vi "GetSensorValues.vi"(1 "Ref_BuiltInAccelerometer":T3={"DevStatus"={"status"=FALSE, "code"=0, "source"=""}, "Scaling"={"Gain (VoltsPerG)"=0.0, "Center Voltage"=0.0}, "Analog Channels"={"X-Axis"=enum."Invalid", "Y-Axis"=enum."Invalid", "Z-Axis"=enum."Invalid"}, "I2C Bus"=enum."Invalid", "SPI Bus"=enum."Invalid", "Accel Range"=0, "ADXL Axes"={"X-Axis"=FALSE, "Y-Axis"=FALSE, "Z-Axis"=FALSE}, "Handle"=0, "Device Address"=0, "Accel Type"=enum."Analog"} {"Device Address" format="%.0x"; "Accel Range" items=["+/- 2 g", "+/- 4 g", "+/- 8 g", "+/- 16 g"]}, 3 "Rear Prox Sensor":T1, 4 "Right Prox Sensor":T1, 5 "Left Prox Sensor":T1, 6 "Upper Pressure Transducer":T1, 8 "Ref_Compressor":T15, 9 "Front-Right Prox Sensor":T1, 10 "Ref_ElevatorEncoder":T10={"DeviceStatus"={"status"=FALSE, "code"=0, "source"=""}, "Type"=enum."PWM", "PWM"={"PWM Channel"=enum."Invalid", "DeadBand"={"Name"="", "maxPositivePwm"=0, "minPositivePwm"=0, "centerPwm"=0, "maxNegativePwm"=0, "minNegativePwm"=0, "angularRange"=0}}, "CAN"={"Device Number"=0, "SetOutput VI Ref"=variant, "GetOutput VI Ref"=variant, "Enable VI Ref"=variant, "Disable VI Ref"=variant, "Data"=variant}, "Invert"=FALSE, "DIO PWM"={"PWM \"Enable\" Channel"=enum."Invalid", "DIOChannel"=enum."Invalid", "PWM Rate"=0.0}}, 11 "Front-Left Prox Sensor":T1, 12 "Ref_ElevatorLimitSwitches":T10={"DeviceStatus"={"status"=FALSE, "code"=0, "source"=""}, "Type"=enum."PWM", "PWM"={"PWM Channel"=enum."Invalid", "DeadBand"={"Name"="", "maxPositivePwm"=0, "minPositivePwm"=0, "centerPwm"=0, "maxNegativePwm"=0, "minNegativePwm"=0, "angularRange"=0}}, "CAN"={"Device Number"=0, "SetOutput VI Ref"=variant, "GetOutput VI Ref"=variant, "Enable VI Ref"=variant, "Disable VI Ref"=variant, "Data"=variant}, "Invert"=FALSE, "DIO PWM"={"PWM \"Enable\" Channel"=enum."Invalid", "DIOChannel"=enum."Invalid", "PWM Rate"=0.0}}, 15 "Tank Pressure Transducer":T1, 19 "Ground Prox Sensor":T1, 20 "Ref_Drive 1R":T10, 21 "Ref_Drive 2R":T10, 22 "Ref_Drive 3L":T10, 23 "Ref_Drive 4L":T10) -> ()   [LabVIEW 2018]
uses:
  <vilib>/Rock Robotics/WPI/AnalogChannel/WPI_AnalogChannelDevRef.ctl
  <vilib>/Rock Robotics/SystemInterfaces/AI/FPGA_AIChannel.ctl
  <vilib>/Rock Robotics/WPI/Compressor/WPI_CompressorDevRef.ctl
  <vilib>/Rock Robotics/WPI/MotorControl/WPI_MotorControlDeviceRef.ctl
  <vilib>/Rock Robotics/WPI/MotorControl/WPI_MotorControlType.ctl
  <vilib>/Rock Robotics/SystemInterfaces/DIO/FPGA_DIOPWMChannel.ctl
  <vilib>/Rock Robotics/WPI/PWM/WPI_PWMDeadband.ctl
  <vilib>/Rock Robotics/SystemInterfaces/DIO/FPGA_DIOChannel.ctl
  <vilib>/Rock Robotics/WPI/Accelerometer/WPI_AccelerometerDevRef.ctl
  <vilib>/Rock Robotics/WPI/Accelerometer/WPI_AccelerometerScaling.ctl
  <vilib>/Rock Robotics/WPI/Accelerometer/WPI_AccelerometerAnalogChannels.ctl
  <vilib>/Rock Robotics/SystemInterfaces/i2clib/i2c_bus.ctl
  <vilib>/Rock Robotics/SystemInterfaces/spilib/spi_bus.ctl
  <vilib>/Rock Robotics/WPI/Accelerometer/ADXL345 Range.ctl
  <vilib>/Rock Robotics/WPI/Accelerometer/WPI_AccelerometerADXL345 Axes.ctl
  SensorReadings.vi
  RefNums_Actuators.vi
  RobotStates.vi
  Inputs_DriverStation.vi
  <vilib>/Rock Robotics/WPI/ThirdParty/Phoenix-LabVIEW/Motor Controller/Get/CTRE_Phoenix_MotorController_GetLimitSwitchStates.vi
  <vilib>/Rock Robotics/WPI/ThirdParty/Phoenix-LabVIEW/Motor Controller/Get/CTRE_Phoenix_MotorController_GetSelectedSensorData.vi
  <vilib>/gmath/NI_Gmath.lvlib
  <vilib>/Analysis/NI_AALBase.lvlib
panel:
  in  "Normal Elevator Std (A)":dbl=35.0
  in  "Off Ground Time (ms)":u32=100
  in  "On Ground Time (ms)":u32=1000
  in  "Ground Distance (in)":dbl=6.0
  in  "Plot Drive Encoder Data":bool
  in  "Tank Pressure Voltage Table":dbl[](array[numeric])=[0.4, 0.7, 0.9, 1.2, 1.4, 1.7, 1.9, 2.3, 2.5, 2.8, 3.0, 3.3] format="%_6g"
  in  "Tank Pressure PSI Table":dbl[](array[numeric])=[0.0, 10.0, 20.0, 30.0, 40.0, 50.0, 60.0, 70.0, 80.0, 90.0, 100.0, 115.0] format="%_6g"
  in  "LR Voltage Table":dbl[](array[numeric])=[0.43, 0.45, 0.47, 0.55, 0.6, 0.68, 0.72, 0.81, 0.86, 0.98, 1.13, 1.36, 1.53, 1.77, 1.99, 2.26, 2.52, 2.76] format="%_6g"
  in  "LR Distance Table":dbl[](array[numeric])=[150.661, 140.6, 133.7, 120.9, 110.1, 95.3, 90.1, 80.0, 73.7, 64.6, 55.9, 45.6, 40.2, 35.0, 29.6, 24.3, 19.6, 14.8] format="%_6g"
  in  "Suction Threshold (V)":dbl=0.15
  in  "SR Voltage Table":dbl[](array[numeric])=[3.15, 2.82, 2.51, 2.16, 1.92, 1.7, 1.49, 1.3, 1.12, 0.97, 0.87, 0.79, 0.72, 0.64, 0.61, 0.58, 0.52, 0.47, 0.46, 0.45, 0.43, 0.41] format="%_6g"
  in  "SR Distance Table":dbl[](array[numeric])=[4.6, 6.6, 8.3, 10.4, 12.2, 14.1, 16.5, 19.9, 23.6, 28.2, 32.6, 36.8, 40.9, 46.3, 49.9, 53.7, 58.3, 63.5, 67.5, 71.5, 75.1, 78.9] format="%_6g"
  out "Drive Encoder Velocities":cluster{dbl, dbl}(graph)
  # "*** Alpha was set to 6 inches ***"
  # "*** Beta was set to 12 inches ***"
  # "ADXL"
  # "Analog"
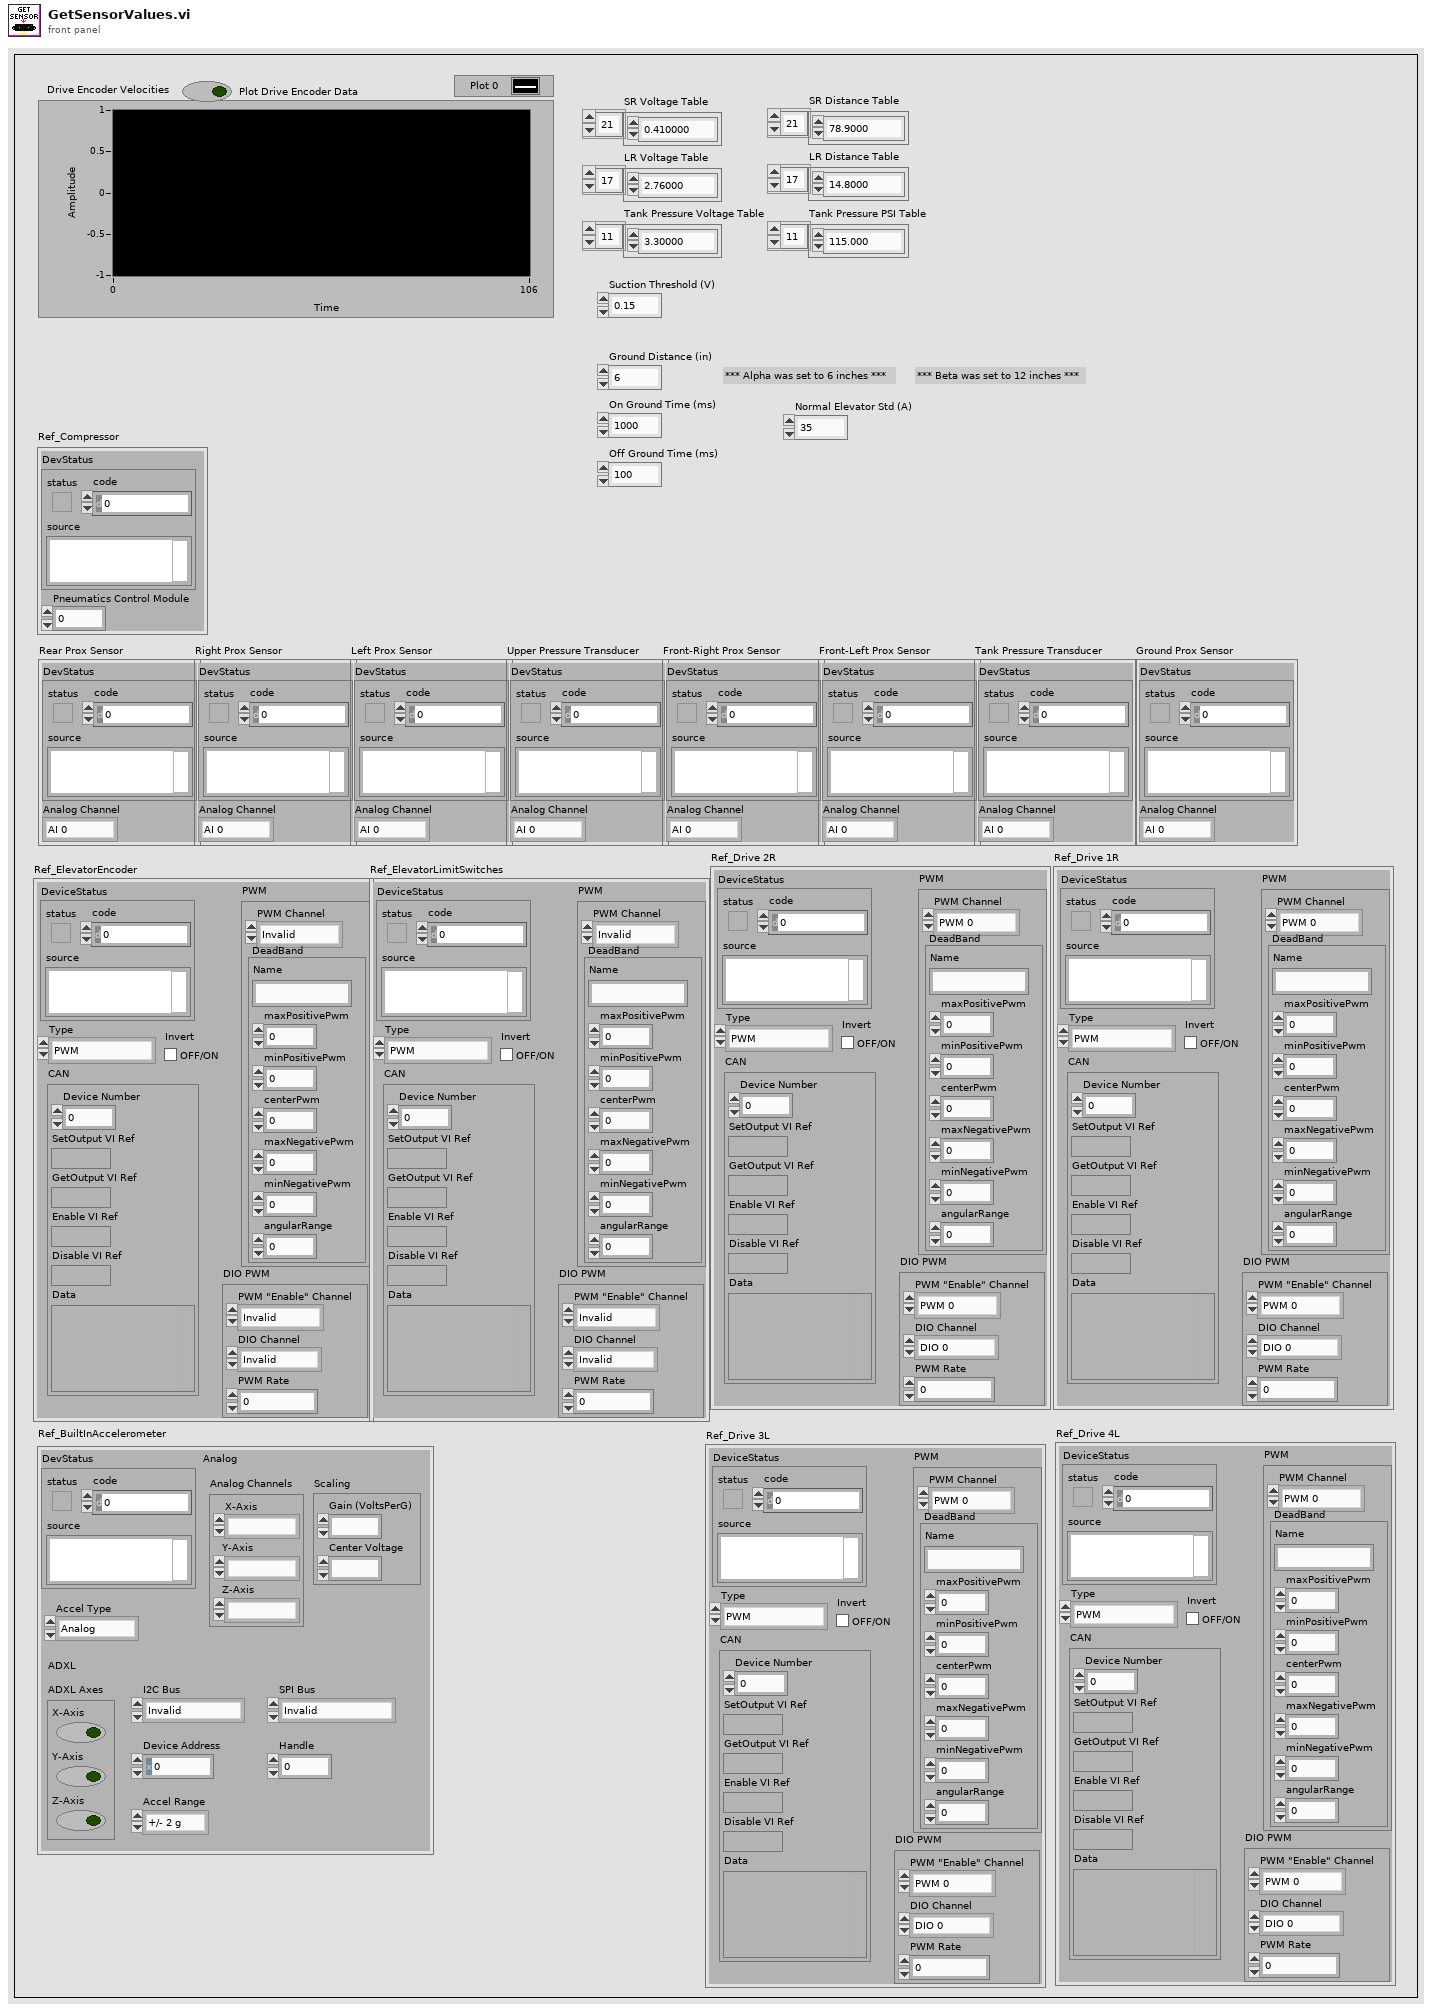
[diagram p1: front panel]
types:
  T1 = typedef "WPI_AnalogChannelDevRef.ctl" = cluster{"DevStatus":errorcluster, "Analog Channel":T2}
  T2 = typedef "FPGA_AIChannel.ctl" = enum8{"AI 0", "AI 1", "AI 2", "AI 3", "AI MXP 0", "AI MXP 1", "AI MXP 2", "AI MXP 3", "Invalid"}
  T3 = typedef "WPI_AccelerometerDevRef.ctl" = cluster{"DevStatus":errorcluster, "Scaling":T4, "Analog Channels":T5, "I2C Bus":T6, "SPI Bus":T7, "Accel Range":T8, "ADXL Axes":T9, "Handle":i32, "Device Address":u8, "Accel Type":enum16{"Analog", "ADXL345 I2C", "ADXL345 SPI", "Internal", "ADXL362 SPI"}}
  T4 = typedef "WPI_AccelerometerScaling.ctl" = cluster{"Gain (VoltsPerG)":dbl, "Center Voltage":dbl}
  T5 = typedef "WPI_AccelerometerAnalogChannels.ctl" = cluster{"X-Axis":T2, "Y-Axis":T2, "Z-Axis":T2}
  T6 = typedef "i2c_bus.ctl" = enum16{"I2C On-Board", "I2C MXP", "Invalid"}
  T7 = typedef "spi_bus.ctl" = enum16{"SPI On-Board, CS0", "SPI On-Board, CS1", "SPI On-Board, CS2", "SPI On-Board, CS3", "SPI MXP", "Invalid"}
  T8 = typedef "ADXL345 Range.ctl" = u8
  T9 = typedef "WPI_AccelerometerADXL345 Axes.ctl" = cluster{"X-Axis":bool, "Y-Axis":bool, "Z-Axis":bool}
  T10 = typedef "WPI_MotorControlDeviceRef.ctl" = cluster{"DeviceStatus":errorcluster, "Type":T11, "PWM":cluster{"PWM Channel":T12, "DeadBand":T13}, "CAN":cluster{"Device Number":u8, "SetOutput VI Ref":variant, "GetOutput VI Ref":variant, "Enable VI Ref":variant, "Disable VI Ref":variant, "Data":variant}, "Invert":bool, "DIO PWM":cluster{"PWM \"Enable\" Channel":T12, "DIOChannel":T14, "PWM Rate":dbl}}
  T11 = typedef "WPI_MotorControlType.ctl" = enum16{"PWM", "CAN", "DIO PWM"}
  T12 = typedef "FPGA_DIOPWMChannel.ctl" = enum8{"PWM 0", "PWM 1", "PWM 2", "PWM 3", "PWM 4", "PWM 5", "PWM 6", "PWM 7", "PWM 8", "PWM 9", "PWM MXP 0", "PWM MXP 1", "PWM MXP 2", "PWM MXP 3", "PWM MXP 4", "PWM MXP 5", "PWM MXP 6", "PWM MXP 7", "PWM MXP 8", "PWM MXP 9", "Invalid"}
  T13 = typedef "WPI_PWMDeadband.ctl" = cluster{"Name":string, "maxPositivePwm":i32, "minPositivePwm":i32, "centerPwm":i32, "maxNegativePwm":i32, "minNegativePwm":i32, "angularRange":u16}
  T14 = typedef "FPGA_DIOChannel.ctl" = enum8{"DIO 0", "DIO 1", "DIO 2", "DIO 3", "DIO 4", "DIO 5", "DIO 6", "DIO 7", "DIO 8", "DIO 9", "DIO MXP 0", "DIO MXP 1", "DIO MXP 2", "DIO MXP 3", "DIO MXP 4", "DIO MXP 5", "DIO MXP 6", "DIO MXP 7", "DIO MXP 8", "DIO MXP 9", "DIO MXP 10", "DIO MXP 11", "DIO MXP 12", "DIO MXP 13", "DIO MXP 14", "DIO MXP 15", "SPI Port CS1", "SPI Port CS2", "SPI Port CS3", "SPI Port MISO", "SPI Port MOSI", "Invalid"}
  T15 = typedef "WPI_CompressorDevRef.ctl" = cluster{"DevStatus":errorcluster, "Pneumatics Control Module":u8}
  T16 = cluster{"X-Axis":dbl, "Y-Axis":dbl, "Z-Axis":dbl}
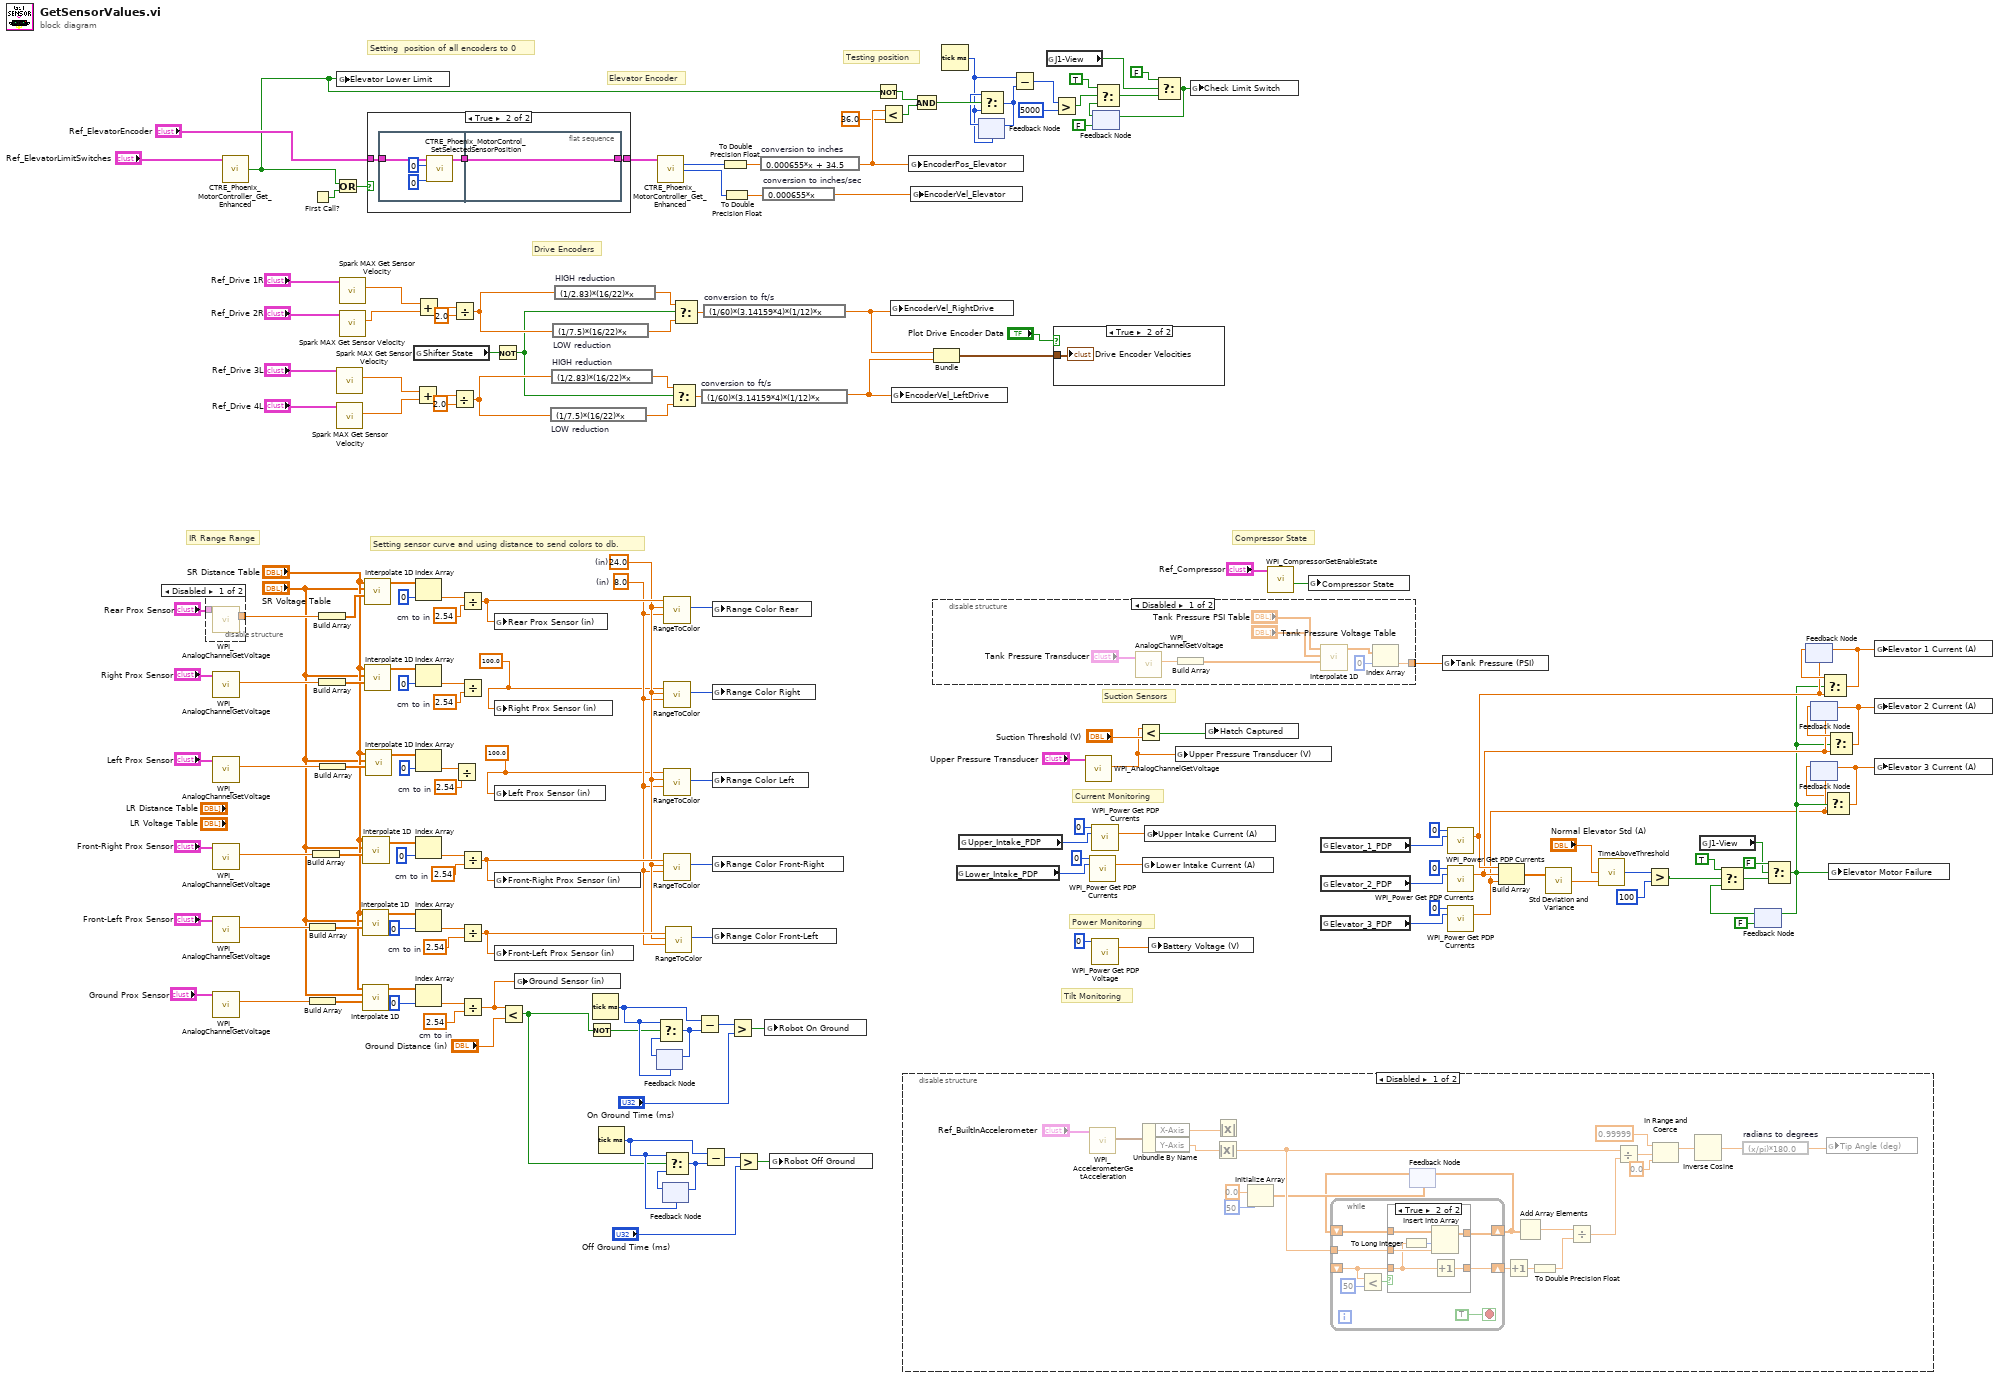
[diagram p0: block diagram]
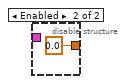
[diagram p2: hidden frame]
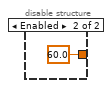
[diagram p6: hidden frame]
diagram:
  w1 = 100.0
  w2 = 100.0
  w72 = 2.54  # cm to in
  w129 = 2.54  # cm to in
  w122 = 8.0  # (in)
  w123 = 24.0  # (in)
  w146 = 2.54  # cm to in
  w152 = 2.54  # cm to in
  w159 = 2.54  # cm to in
  w166 = 2.54  # cm to in
  # "Elevator Encoder"
  # "Tilt Monitoring"
  # "Drive Encoders"
  # "Power Monitoring"
  # "Testing position"
  # "Setting  position of all encoders to 0"
  # "Setting sensor curve and using distance to send colors to db."
  # "Current Monitoring"
  # "Suction Sensors"
  # "Compressor State"
  # "IR Range Range"
  n1 = disable-structure shown="Disabled" {
    disable-tunnel: [w172 0.0 ("Voltage")] -> w170
    disable-tunnel: "Rear Prox Sensor" -> [w171 _]
    frame Disabled {
      n2 = call <vilib>:"WPI_AnalogChannelGetVoltage.vi"("AIDeviceRef"=w171) -> ("Voltage"=w172:dbl)  [unwired: 8 in, 2 out]
    }
    frame Enabled {
    }
  }
  n3 = call <vilib>:"WPI_AnalogChannelGetVoltage.vi"("AIDeviceRef"="Right Prox Sensor") -> ("Voltage"=w164:dbl)  [unwired: 8 in, 2 out]
  n4 = call <vilib>:"WPI_AnalogChannelGetVoltage.vi"("AIDeviceRef"="Left Prox Sensor") -> ("Voltage"=w157:dbl)  [unwired: 8 in, 2 out]
  n5 = call <vilib>:"WPI_AnalogChannelGetVoltage.vi"("AIDeviceRef"="Front-Right Prox Sensor") -> ("Voltage"=w134:dbl)  [unwired: 8 in, 2 out]
  n6 = call <vilib>:"WPI_AnalogChannelGetVoltage.vi"("AIDeviceRef"="Front-Left Prox Sensor") -> ("Voltage"=w127:dbl)  [unwired: 8 in, 2 out]
  n7 = call <vilib>:"WPI_AnalogChannelGetVoltage.vi"("AIDeviceRef"="Ground Prox Sensor") -> ("Voltage"=w71:dbl)  [unwired: 8 in, 2 out]
  n8 = call-poly <vilib>:"CTRE_Phoenix_MotorController_Get_Enhanced.vi"("PhoenixMotorControlDevRef"="Ref_ElevatorLimitSwitches") -> ("Reverse Limit Closed?"=w18:bool)  [unwired: 11 in, 3 out]
  n9 = First Call?() -> (First Call?: T/F=w76:bool)
  n10 = Build Array(w127) -> (w132:dbl[])
  n11 = Build Array(w71) -> (w75:dbl[])
  n12 = Build Array(w134) -> (w150:dbl[])
  n13 = Build Array(w170) -> (w144:dbl[])
  n14 = Build Array(w164) -> (w163:dbl[])
  n15 = Build Array(w157) -> (w156:dbl[])
  n16 = Or(x=w18, y=w76) -> (x .or. y?=w77:bool)
  n17 = global write "SensorReadings.vi" "Elevator Lower Limit"(w18) -> ()
  n18 = call <vilib>:"Spark MAX Get Sensor Velocity.vi"("MotorControlDevRef in"="Ref_Drive 3L") -> ("Sensor Velocity"=w104:dbl)  [unwired: 7 in, 3 out]
  n19 = call <vilib>:"Spark MAX Get Sensor Velocity.vi"("MotorControlDevRef in"="Ref_Drive 4L") -> ("Sensor Velocity"=w103:dbl)  [unwired: 7 in, 3 out]
  n20 = call <vilib>:"Spark MAX Get Sensor Velocity.vi"("MotorControlDevRef in"="Ref_Drive 1R") -> ("Sensor Velocity"=w109:dbl)  [unwired: 7 in, 3 out]
  n21 = call <vilib>:"Spark MAX Get Sensor Velocity.vi"("MotorControlDevRef in"="Ref_Drive 2R") -> ("Sensor Velocity"=w50:dbl)  [unwired: 7 in, 3 out]
  n22 = call <vilib>:"Interpolate 1D.vi"("xi"=w132, "X"="SR Voltage Table", "Y"="SR Distance Table") -> ("yi"=w126:dbl[])  [unwired: 6 in, 2 out]
  n23 = call <vilib>:"Interpolate 1D.vi"("xi"=w75, "X"="SR Voltage Table", "Y"="SR Distance Table") -> ("yi"=w70:dbl[])  [unwired: 6 in, 2 out]
  n24 = call <vilib>:"Interpolate 1D.vi"("xi"=w150, "X"="SR Voltage Table", "Y"="SR Distance Table") -> ("yi"=w147:dbl[])  [unwired: 6 in, 2 out]
  n25 = call <vilib>:"Interpolate 1D.vi"("xi"=w144, "X"="SR Voltage Table", "Y"="SR Distance Table") -> ("yi"=w167:dbl[])  [unwired: 6 in, 2 out]
  n26 = call <vilib>:"Interpolate 1D.vi"("xi"=w163, "X"="SR Voltage Table", "Y"="SR Distance Table") -> ("yi"=w160:dbl[])  [unwired: 6 in, 2 out]
  n27 = call <vilib>:"Interpolate 1D.vi"("xi"=w156, "X"="SR Voltage Table", "Y"="SR Distance Table") -> ("yi"=w153:dbl[])  [unwired: 6 in, 2 out]
  n28 = case shown="True" w77 {
    tunnel: "Ref_ElevatorEncoder" -> [w174 w177]
    tunnel: [w174 w175] -> w82
    frame False {
    }
    frame True {
      n29 = flat-sequence {
        tunnel: w177 -> [w181]
        tunnel: [w180] -> w176
        tunnel: [w182] -> w175
        tunnel: w176 -> [w182]
        frame #0 {
          n30 = call <vilib>:"CTRE_Phoenix_MotorControl_SetSelectedSensorPosition.vi"("pidLoopIdx"=u32 0, "New Sensor Position"=0, "PhoenixMotorControlDevRef"=w181) -> ("PhoenixMotorControlDevRef"=w180:T10)  [unwired: 7 in, 1 out]
        }
        frame #1 {
        }
      }
    }
  }
  n31 = global read "RobotStates.vi" "Shifter State"() -> (w96:bool)
  n32 = Add(x=w104, y=w103) -> (x+y=w106:dbl)
  n33 = Add(x=w109, y=w50) -> (x+y=w108:dbl)
  n34 = Index Array(array=w167, index=0) -> (element=w168:dbl)
  n35 = Index Array(array=w160, index=0) -> (element=w161:dbl)
  n36 = Index Array(array=w153, index=0) -> (element=w154:dbl)
  n37 = Index Array(array=w147, index=0) -> (element=w148:dbl)
  n38 = Index Array(array=w126, index=0) -> (element=w130:dbl)
  n39 = Index Array(array=w70, index=0) -> (element=w73:dbl)
  n40 = Divide(x=w106, y=2.0) -> (x/y=w97:dbl)
  n41 = Divide(x=w108, y=2.0) -> (x/y=w100:dbl)
  n42 = Divide(x=w154, y=w152) -> ()  [unwired: 1 out]
  n43 = Divide(x=w168, y=w166) -> (x/y=w143:dbl)
  n44 = Divide(x=w161, y=w159) -> ()  [unwired: 1 out]
  n45 = Divide(x=w148, y=w146) -> (x/y=w142:dbl)
  n46 = Divide(x=w130, y=w129) -> (x/y=w128:dbl)
  n47 = Divide(x=w73, y=w72) -> (x/y=w53:dbl)
  n48 = Not(x=w96) -> (.not. x?=w84:bool)
  n49 = global write "SensorReadings.vi" "Rear Prox Sensor (in)"(w143) -> ()
  n50 = global write "SensorReadings.vi" "Right Prox Sensor (in)"(w2) -> ()
  n51 = global write "SensorReadings.vi" "Left Prox Sensor (in)"(w1) -> ()
  n52 = global write "SensorReadings.vi" "Front-Right Prox Sensor (in)"(w142) -> ()
  n53 = global write "SensorReadings.vi" "Front-Left Prox Sensor (in)"(w128) -> ()
  n54 = Less?(x=w53, y="Ground Distance (in)") -> (x < y?=w52:bool)
  n55 = global write "SensorReadings.vi" "Ground Sensor (in)"(w53) -> ()
  n56 = expression code="(1/7.5)*(16/22)*x" "LOW reduction"(w97) -> (w98:dbl)
  n57 = expression code="(1/2.83)*(16/22)*x" "HIGH reduction"(w97) -> (w99:dbl)
  n58 = expression code="(1/7.5)*(16/22)*x" "LOW reduction"(w100) -> (w101:dbl)
  n59 = expression code="(1/2.83)*(16/22)*x" "HIGH reduction"(w100) -> (w102:dbl)
  n60 = Not(x=w52) -> (.not. x?=w51:bool)
  n61 = Tick Count (ms)() -> (millisecond timer value=w63:u32)
  n62 = Tick Count (ms)() -> (millisecond timer value=w58:u32)
  n63 = feedback #1(w63) -> (w65:u32)
  n64 = call-poly <vilib>:"CTRE_Phoenix_MotorController_Get_Enhanced.vi"("PhoenixMotorControlDevRef"=w82) -> ("Position (Raw Sensor Units)"=w81:i32, "Velocity (Raw Sensor Units per 100 ms)"=w79:i32)  [unwired: 11 in, 2 out]
  n65 = Select(t=w63, s=w51, f=w65) -> (s? t:f=w64:u32)
  n66 = feedback-in #1(w64) -> ()
  n67 = feedback #2(w58) -> (w60:u32)
  n68 = call "RangeToColor.vi"("Really Close (in)"=w122, "Close (in)"=w123, "Range (in)"=w143) -> ("Range Color"=w141:u32)  [unwired: 8 in]
  n69 = call "RangeToColor.vi"("Really Close (in)"=w122, "Close (in)"=w123, "Range (in)"=w2) -> ("Range Color"=w140:u32)  [unwired: 8 in]
  n70 = call "RangeToColor.vi"("Really Close (in)"=w122, "Close (in)"=w123, "Range (in)"=w1) -> ("Range Color"=w139:u32)  [unwired: 8 in]
  n71 = call "RangeToColor.vi"("Really Close (in)"=w122, "Close (in)"=w123, "Range (in)"=w142) -> ("Range Color"=w138:u32)  [unwired: 8 in]
  n72 = Select(t=w58, s=w52, f=w60) -> (s? t:f=w59:u32)
  n73 = feedback-in #2(w59) -> ()
  n74 = call "RangeToColor.vi"("Really Close (in)"=w122, "Close (in)"=w123, "Range (in)"=w128) -> ("Range Color"=w124:u32)  [unwired: 8 in]
  n75 = Select(t=w99, s=w84, f=w98) -> (s? t:f=w86:dbl)
  n76 = Select(t=w102, s=w84, f=w101) -> (s? t:f=w88:dbl)
  n77 = Subtract(x=w63, y=w64) -> (x-y=w62:u32)
  n78 = expression code="(1/60)*(3.14159*4)*(1/12)*x" "conversion to ft/s"(w86) -> (w85:dbl)
  n79 = Subtract(x=w58, y=w59) -> (x-y=w57:u32)
  n80 = expression code="(1/60)*(3.14159*4)*(1/12)*x" "conversion to ft/s"(w88) -> (w87:dbl)
  n81 = global write "SensorReadings.vi" "Range Color Rear"(w141) -> ()
  n82 = global write "SensorReadings.vi" "Range Color Right"(w140) -> ()
  n83 = global write "SensorReadings.vi" "Range Color Left"(w139) -> ()
  n84 = global write "SensorReadings.vi" "Range Color Front-Right"(w138) -> ()
  n85 = global write "SensorReadings.vi" "Range Color Front-Left"(w124) -> ()
  n86 = To Double Precision Float(number=w81) -> (double precision float=w83:dbl)
  n87 = To Double Precision Float(number=w79) -> (double precision float=w80:dbl)
  n88 = Greater?(x=w62, y="On Ground Time (ms)") -> (0:w61:bool)
  n89 = Greater?(x=w57, y="Off Ground Time (ms)") -> (0:w56:bool)
  n90 = expression code="0.000655*x + 34.5" "conversion to inches"(w83) -> (w21:dbl)
  n91 = expression code="0.000655*x" "conversion to inches/sec"(w80) -> (w78:dbl)
  n92 = global write "SensorReadings.vi" "Robot On Ground"(w61) -> ()
  n93 = global write "SensorReadings.vi" "Robot Off Ground"(w56) -> ()
  n94 = Not(x=w18) -> (.not. x?=w20:bool)
  n95 = Less?(x=w21, y=36.0) -> (x < y?=w19:bool)
  n96 = global write "SensorReadings.vi" "EncoderVel_RightDrive"(w87) -> ()
  n97 = global write "SensorReadings.vi" "EncoderVel_LeftDrive"(w85) -> ()
  n98 = disable-structure shown="Disabled" {
    frame Disabled {
      n99 = call <vilib>:"WPI_AccelerometerGetAcceleration.vi"("AccelerometerDevRef"="Ref_BuiltInAccelerometer") -> ("Accelerations"=w203:T16)  [unwired: 8 in, 2 out]
      n100 = Unbundle By Name(w203) -> ("X-Axis"=w201:dbl, "Y-Axis"=w200:dbl)
      n101 = Absolute Value(x=w200) -> (abs(x)=w191:dbl)
      n102 = Absolute Value(x=w201) -> ()  [unwired: 1 out]
      n103 = Initialize Array(0.0 ("element"), 50 ("dimension size")) -> (w188:dbl[])
      n104 = feedback #3(w188) -> (w187:dbl[])
      n105 = while {
        shift-right: [w209] -> w189
        shift-left: w187 -> [w210]
        tunnel: w191 -> [w204]
        shift-right: [w208] -> w194
        shift-left: _ -> [w206]
        stop <- TRUE stop-if-true
        n106 = Less?(x=w206, y=50) -> (x < y?=w207:bool)
        n107 = case shown="True" w207 {
          tunnel: w210 -> [w213 w219]
          tunnel: [w213 w218] -> w209
          tunnel: w204 -> [_ w217]
          tunnel: w206 -> [w212 w216]
          tunnel: [w212 w215] -> w208
          frame False {
          }
          frame True {
            n108 = To Long Integer(number=w216) -> (32bit integer=w214:i32)
            n109 = Insert Into Array(array=w219, index=w214, new element=w217) -> (w218:dbl[])
            n110 = Increment(x=w216) -> (x+1=w215:dbl)
          }
        }
      }
      n111 = feedback-in #3(w189) -> ()
      n112 = Increment(x=w194) -> (x+1=w193:dbl)
      n113 = Add Array Elements(numeric array=w189) -> (sum=w195:dbl)
      n114 = To Double Precision Float(number=w193) -> (double precision float=w192:dbl)
      n115 = Divide(x=w195, y=w192) -> (x/y=w190:dbl)
      n116 = Divide(x=w191, y=w190) -> (x/y=w186:dbl)
      n117 = In Range and Coerce(upper limit=0.99999, x=w186, lower limit=0.0) -> (coerced(x)=w185:dbl)  [unwired: 1 out]
      n118 = Inverse Cosine(1:w185) -> (0:w198:dbl)
      n119 = expression code="(x/pi)*180.0" "radians to degrees"(w198) -> (w199:dbl)
      n120 = global write "SensorReadings.vi" "Tip Angle (deg)"(w199) -> ()
    }
    frame Enabled {
    }
  }
  n121 = global write "SensorReadings.vi" "EncoderPos_Elevator"(w21) -> ()
  n122 = global write "SensorReadings.vi" "EncoderVel_Elevator"(w78) -> ()
  n123 = Compound Arithmetic op=AND(w20, w19) -> (w11:bool)
  n124 = disable-structure shown="Disabled" {
    disable-tunnel: [w221 60.0 ("Tank Pressure (PSI)")] -> w114
    frame Disabled {
      n125 = call <vilib>:"WPI_AnalogChannelGetVoltage.vi"("AIDeviceRef"="Tank Pressure Transducer") -> ("Voltage"=w220:dbl)  [unwired: 8 in, 2 out]
      n126 = Build Array(w220) -> (w222:dbl[])
      n127 = call <vilib>:"Interpolate 1D.vi"("xi"=w222, "X"="Tank Pressure Voltage Table", "Y"="Tank Pressure PSI Table") -> ("yi"=w225:dbl[])  [unwired: 6 in, 2 out]
      n128 = Index Array(array=w225, index=0) -> (element=w221:dbl)
    }
    frame Enabled {
    }
  }
  n129 = Bundle(w87, w85) -> (w95:cluster{dbl, dbl})  [unwired: 1 in]
  n130 = Tick Count (ms)() -> (millisecond timer value=w5:u32)
  n131 = global read "RefNums_Actuators.vi" "Lower_Intake_PDP"() -> (w117:i32)
  n132 = global read "RefNums_Actuators.vi" "Upper_Intake_PDP"() -> (w120:i32)
  n133 = feedback #4(w5) -> (w10:u32)
  n134 = Select(t=w10, s=w11, f=w5) -> (s? t:f=w6:u32)
  n135 = feedback-in #4(w6) -> ()
  n136 = Subtract(x=w5, y=w6) -> (x-y=w4:u32)
  n137 = global read "Inputs_DriverStation.vi" "J1-View"() -> (w12:bool)
  n138 = Greater?(x=w4, y=u32 5000) -> (0:w7:bool)
  n139 = case shown="True" "Plot Drive Encoder Data" {
    tunnel: w95 -> [_ w229]
    frame False {
    }
    frame True {
      "Drive Encoder Velocities" <- w229
    }
  }
  n140 = call <vilib>:"WPI_AnalogChannelGetVoltage.vi"("AIDeviceRef"="Upper Pressure Transducer") -> ("Voltage"=w115:dbl)  [unwired: 8 in, 2 out]
  n141 = call <vilib>:"WPI_Power Get PDP Currents.vi"("Power Distribution Panel (0)"=u8 0, "PDP Channel"=w117) -> ("current (A)"=w116:dbl)  [unwired: 11 in, 2 out]
  n142 = call <vilib>:"WPI_Power Get PDP Currents.vi"("Power Distribution Panel (0)"=u8 0, "PDP Channel"=w120) -> ("current (A)"=w119:dbl)  [unwired: 11 in, 2 out]
  n143 = call <vilib>:"WPI_Power Get PDP Voltage.vi"("Power Distribution Panel (0)"=u8 0) -> ("voltage (V)"=w112:dbl)  [unwired: 13 in, 1 out]
  n144 = feedback #5(FALSE) -> (w17:bool)
  n145 = Select(t=TRUE, s=w7, f=w17) -> (s? t:f=w14:bool)
  n146 = Less?(x=w115, y="Suction Threshold (V)") -> (x < y?=w89:bool)
  n147 = global write "SensorReadings.vi" "Lower Intake Current (A)"(w116) -> ()
  n148 = global write "SensorReadings.vi" "Upper Intake Current (A)"(w119) -> ()
  n149 = global write "SensorReadings.vi" "Battery Voltage (V)"(w112) -> ()
  n150 = Select(t=FALSE, s=w12, f=w14) -> (s? t:f=w3:bool)
  n151 = feedback-in #5(w3) -> ()
  n152 = global write "SensorReadings.vi" "Upper Pressure Transducer (V)"(w115) -> ()
  n153 = global write "RobotStates.vi" "Check Limit Switch"(w3) -> ()
  n154 = global write "SensorReadings.vi" "Hatch Captured"(w89) -> ()
  n155 = call <vilib>:"WPI_CompressorGetEnableState.vi"("CompressorDevRef"="Ref_Compressor") -> ("Compressor Running"=w136:bool)  [unwired: 7 in, 3 out]
  n156 = global write "RobotStates.vi" "Compressor State"(w136) -> ()
  n157 = global read "RefNums_Actuators.vi" "Elevator_1_PDP"() -> (w48:i32)
  n158 = global read "RefNums_Actuators.vi" "Elevator_2_PDP"() -> (w46:i32)
  n159 = global read "RefNums_Actuators.vi" "Elevator_3_PDP"() -> (w44:i32)
  n160 = global write "SensorReadings.vi" "Tank Pressure (PSI)"(w114) -> ()
  n161 = call <vilib>:"WPI_Power Get PDP Currents.vi"("Power Distribution Panel (0)"=u8 0, "PDP Channel"=w48) -> ("current (A)"=w30:dbl)  [unwired: 11 in, 2 out]
  n162 = call <vilib>:"WPI_Power Get PDP Currents.vi"("Power Distribution Panel (0)"=u8 0, "PDP Channel"=w46) -> ("current (A)"=w27:dbl)  [unwired: 11 in, 2 out]
  n163 = call <vilib>:"WPI_Power Get PDP Currents.vi"("Power Distribution Panel (0)"=u8 0, "PDP Channel"=w44) -> ("current (A)"=w24:dbl)  [unwired: 11 in, 2 out]
  n164 = Build Array(w30, w27, w24) -> (w43:dbl[])
  n165 = call <vilib>:"Std Deviation and Variance.vi"("X"=w43) -> ("standard deviation"=w42:dbl)  [unwired: 1 in, 2 out]
  n166 = call "TimeAboveThreshold.vi"("Current Value"=w42, "Threshold"="Normal Elevator Std (A)") -> ("Time Above"=w40:u32)  [unwired: 3 in]
  n167 = Greater?(x=w40, y=u32 100) -> (0:w32:bool)
  n168 = global read "Inputs_DriverStation.vi" "J1-View"() -> (w33:bool)
  n169 = feedback #6(FALSE) -> (w37:bool)
  n170 = Select(t=TRUE, s=w32, f=w37) -> (s? t:f=w35:bool)
  n171 = Select(t=FALSE, s=w33, f=w35) -> (s? t:f=w25:bool)
  n172 = feedback-in #6(w25) -> ()
  n173 = feedback #7(w30) -> (w31:dbl)
  n174 = feedback #8(w27) -> (w28:dbl)
  n175 = feedback #9(w24) -> (w22:dbl)
  n176 = Select(t=w31, s=w25, f=w30) -> (s? t:f=w29:dbl)
  n177 = feedback-in #7(w29) -> ()
  n178 = Select(t=w22, s=w25, f=w24) -> (s? t:f=w23:dbl)
  n179 = feedback-in #9(w23) -> ()
  n180 = Select(t=w28, s=w25, f=w27) -> (s? t:f=w26:dbl)
  n181 = feedback-in #8(w26) -> ()
  n182 = global write "RobotStates.vi" "Elevator Motor Failure"(w25) -> ()
  n183 = global write "SensorReadings.vi" "Elevator 1 Current (A)"(w29) -> ()
  n184 = global write "SensorReadings.vi" "Elevator 2 Current (A)"(w26) -> ()
  n185 = global write "SensorReadings.vi" "Elevator 3 Current (A)"(w23) -> ()
